vi "WriteSignals.Compile.vi"(8 "error in (no error)":errorcluster, 10 "Settings":T4[](array[typedef]) {"Signal.Cmd.Refs"."Signal Refs" format="%.0x"; "Signal.Cmd.Info"."Signals"."Byte Order" items=["Little Endian", "Big Endian"]; "Signal.Cmd.Info"."Signals"."Data Type" items=["Signed", "Unsigned", "IEEE Float"]; "Settings.Refs"."Signal Refs" format="%.0x"; "Signal.Resp.Refs"."Signal Refs" format="%.0x"; "Signal.Resp.Info"."Signals"."Byte Order" items=["Little Endian", "Big Endian"]; "Signal.Resp.Info"."Signals"."Data Type" items=["Signed", "Unsigned", "IEEE Float"]; "Trigger.Refs"."Signal Refs" format="%.0x"; "Status.Refs"."Signal Refs" format="%.0x"}, 11 "Lookup In":variant) -> (0 "error out":errorcluster, 1 "Signal Info":T1[](array[typedef]) {"Signals"."Byte Order" items=["Little Endian", "Big Endian"]; "Signals"."Data Type" items=["Signed", "Unsigned", "IEEE Float"]}, 2 "Refs":T7 {"VS Refs" format="%.0x"}, 3 "Lookup":variant)   [LabVIEW 2019, in "Diagnostics Addon System Explorer.lvlib"]
uses:
  Diagnostics Addon System Explorer.lvlib
  <vilib>/NI VeriStand/Custom Device API/Custom Device Item Ref.ctl
  Types/Service.Export.ctl
  Types/Frame.Ref.ctl
  Addon Shared/Types/Type.ctl
  Addon Shared/Types/Frame.Compile.ctl
  Addon Shared/Types/Signal.ctl
  Addon Shared/Types/Frame.Lookup.Info.ctl
  Addon Shared/SubVIs/Constants.vi
  Addon Shared/Diagnostics Addon Shared.lvlib
  <vilib>/NI VeriStand/Custom Device API/Custom Device API.lvlib
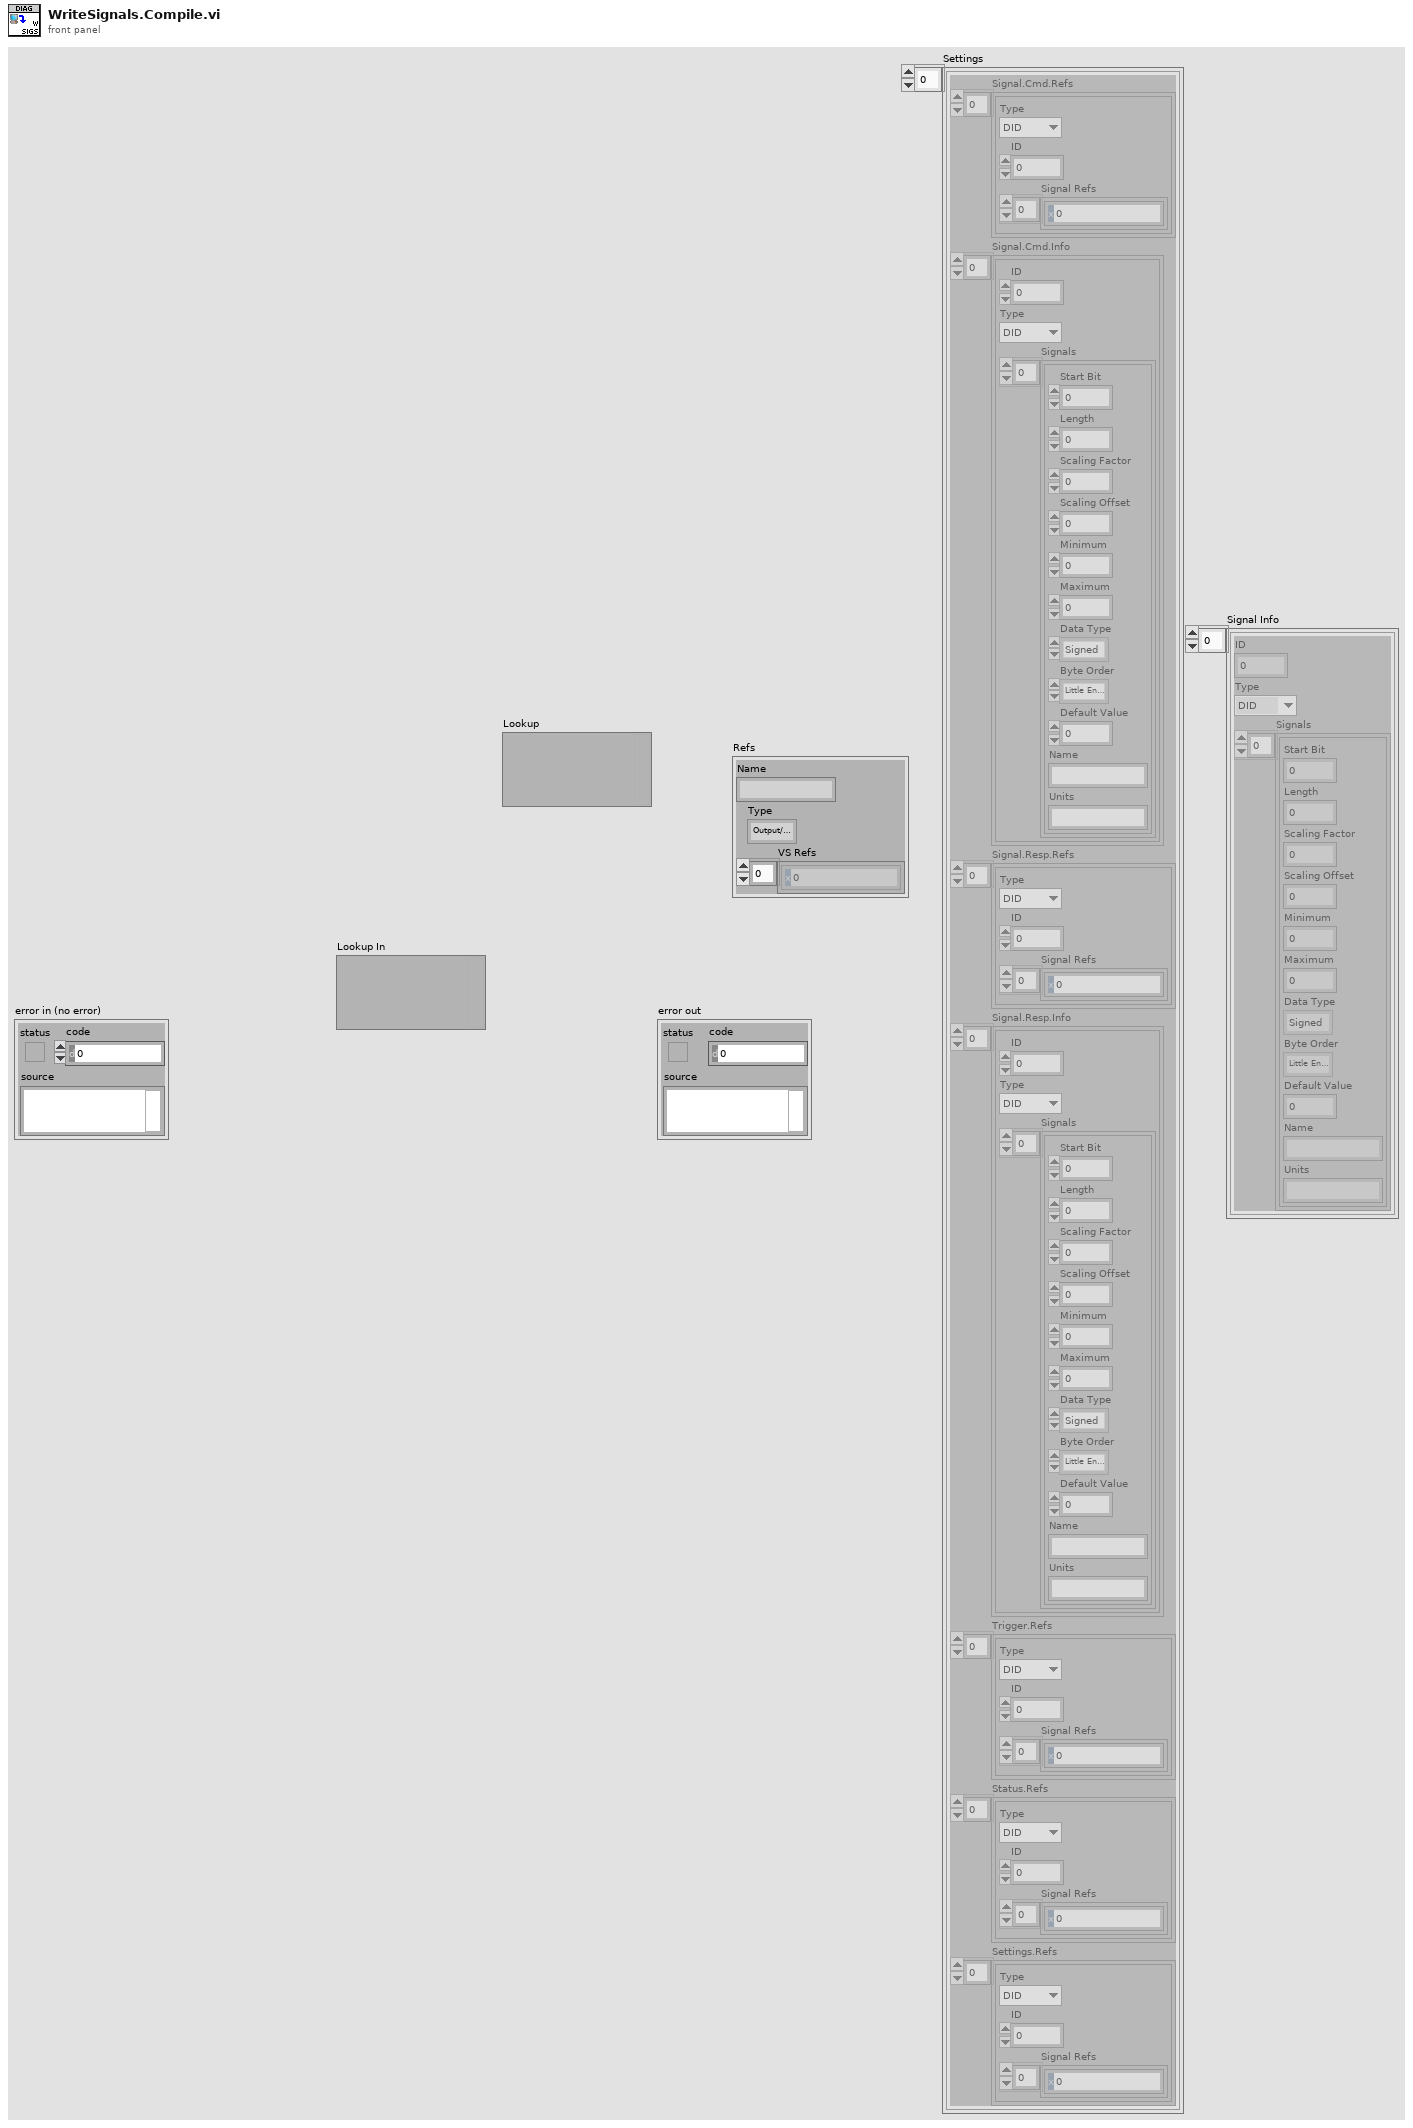
[diagram p1: front panel]
types:
  T1 = typedef "Diagnostics Addon Shared.lvlib/Frame.Compile.ctl" = cluster{"ID":u32, "Type":T2, "Signals":T3[]}
  T2 = typedef "Diagnostics Addon Shared.lvlib/Type.ctl" = enum16{"DID", "CDID", "PID", "CPID", "Read Memory", "Write Memory", "IO Control", "Routine Start", "Routine Request", "Routine Stop", "User Defined", "DTC Control", "Clear DTCs", "Read DTCs", "Start DTCs", "DTC Change Count", "Tester Present", "Unlock ECU", "Reset ECU", "Diag Session Control", "Communication Control", "DPID Control", "Poll Control", "Diag CAN Control"}
  T3 = typedef "Diagnostics Addon Shared.lvlib/Signal.ctl" = cluster{"Start Bit":u32, "Length":u32, "Scaling Factor":dbl, "Scaling Offset":dbl, "Minimum":dbl, "Maximum":dbl, "Data Type":u32, "Byte Order":u32, "Default Value":dbl, "Name":string, "Units":string}
  T4 = typedef "Diagnostics Addon System Explorer.lvlib/Service.Export.ctl" = cluster{"Signal.Cmd.Refs":T5[], "Signal.Cmd.Info":T1[], "Signal.Resp.Refs":T5[], "Signal.Resp.Info":T1[], "Trigger.Refs":T5[], "Status.Refs":T5[], "Settings.Refs":T5[]}
  T5 = typedef "Diagnostics Addon System Explorer.lvlib/Frame.Ref.ctl" = cluster{"Type":T2, "ID":u32, "Signal Refs":T6[]}
  T6 = typedef "Custom Device API.lvlib/Custom Device Item Ref.ctl" = u64
  T7 = cluster{"Name":string, "Type":enum16{"Output/Write", "Input/Read", "Input/ReadWrite"}, "VS Refs":T6[]}
  T8 = enum16{"Output/Write", "Input/Read", "Input/ReadWrite"}
  T9 = typedef "Diagnostics Addon Shared.lvlib/Frame.Lookup.Info.ctl" = cluster{"Offset":i32, "Length":i32, "ByteLength":u16}
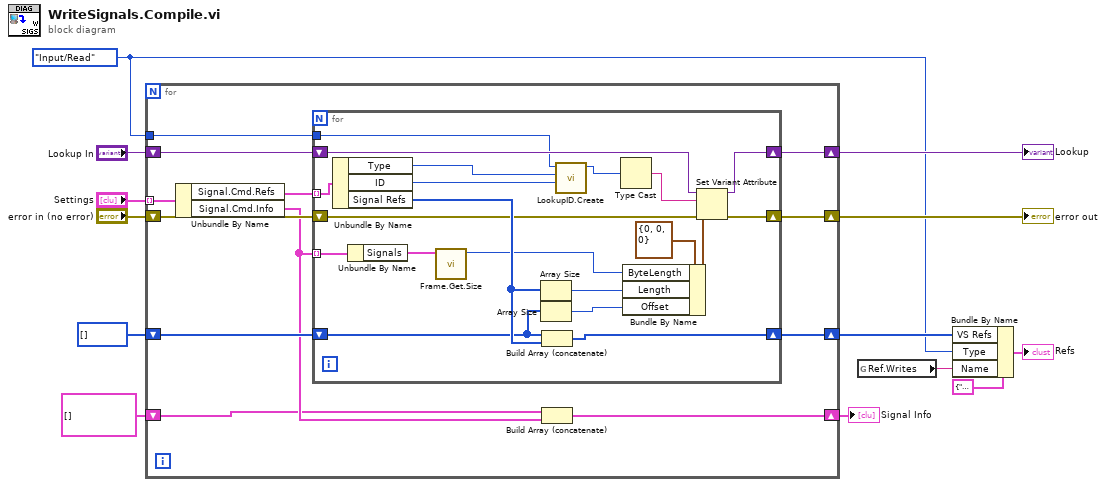
[diagram p0: block diagram]
diagram:
  w1 = T8."Input/Read" ("Type")
  n1 = for {
    shift-right: [w20] -> w5
    shift-left: "error in (no error)" -> [w25]
    shift-right: [w24] -> w12
    shift-left: "Lookup In" -> [w22]
    shift-right: [w21] -> w6
    shift-left: T6[] [] -> [w23]
    tunnel: "Settings" -> [w19] mode=indexing
    shift-right: [w16] -> w2
    shift-left: T1[] [] -> [w15]
    tunnel: w1 -> [w14]
    n2 = Unbundle By Name(w19) -> ("Signal.Cmd.Refs"=w18:T5[], "Signal.Cmd.Info"=w17:T1[])
    n3 = for {
      tunnel: w18 -> [w37] mode=indexing
      shift-right: [w38] -> w24
      shift-left: w22 -> [w42]
      shift-right: [w40] -> w20
      shift-left: w25 -> [w33]
      shift-right: [w36] -> w21
      shift-left: w23 -> [w34]
      tunnel: w17 -> [w32] mode=indexing
      tunnel: w14 -> [w26]
      n4 = Unbundle By Name(w37) -> ("Type"=w28:T2, "ID"=w29:u32, "Signal Refs"=w35:T6[])
      n5 = Unbundle By Name(w32) -> ("Signals"=w31:T3[])
      n6 = call "Frame.Get.Size.vi"("Parameters"=w31) -> ("Bytes"=w30:u32)  [unwired: 10 in]
      n7 = Array Size(array=w35) -> (size(s)=w45:i32)
      n8 = Array Size(array=w34) -> (size(s)=w41:i32)
      n9 = Build Array (concatenate)(w34, w35) -> (w36:T6[])
      n10 = call "LookupID.Create.vi"("Serivce ID"=w29, "Service Type"=w28, "Direction"=w26) -> ("Result"=w27:u64)  [unwired: 8 in]
      n11 = Type Cast(x=w27) -> (*(type *) &x=w39:string)  [unwired: 1 in]
      n12 = Bundle By Name(cluster=T9 {"Offset"=0, "Length"=0, "ByteLength"=0}, "ByteLength"=w30, "Length"=w45, "Offset"=w41) -> (w43:T9)
      n13 = Set Variant Attribute(Variant=w42, name=w39, value=w43, error in=w33) -> (Variant out=w38:variant, error out=w40:errorcluster)  [unwired: 1 out]
    }
    n14 = Build Array (concatenate)(w15, w17) -> (w16:T1[])
  }
  "error out" <- w5
  "Lookup" <- w12
  "Signal Info" <- w2
  n15 = global read "Constants.vi" "Ref.Writes"() -> (w8:string)
  n16 = Bundle By Name(cluster=T7 {"Name"="", "Type"=enum."Output/Write", "VS Refs"=[]} ("Group"), "VS Refs"=w6, "Type"=w1, "Name"=w8) -> (→"Refs":T7)
